vi "global_variable_1.vi"() -> ()   [LabVIEW 2021]
panel:
  in  "Temp_other_mode":bool
  out "is_connected":bool
  in  "vout_iout":string[](array[string])
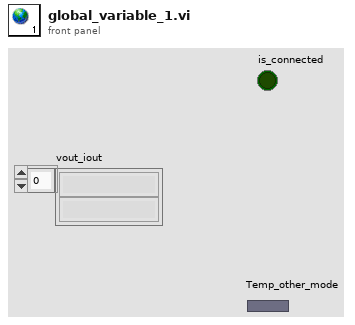
[diagram p1: front panel]
diagram:
